vi "Initialize Sink.vi"(11 "Buffered Log Sink in":refnum<class "Buffered Log Sink.lvclass">) -> (0 "error out":errorcluster, 3 "Buffered Log Sink out":refnum<class "Buffered Log Sink.lvclass">)   [LabVIEW 2020, in "Buffered Log Sink.lvclass"]
uses:
  <vilib>/gpm_packages/@cs/event-logger/Source/Buffered Log Sink/Buffered Log Sink.lvclass
  <vilib>/gpm_packages/@cs/event-logger/Source/Buffered Log Sink/Buffered Log Sink.lvclass/Buffered Log Sink.ctl
  <vilib>/gpm_packages/@cs/event-logger/Source/Composed Log/Types/Log Packet.ctl
  <vilib>/gpm_packages/@cs/event-logger/Source/Composed Log/Types/Log Level.ctl
  <vilib>/gpm_packages/@cs/event-logger/Source/Buffered Log Sink/Timeout Watchdog.vi
  <vilib>/gpm_packages/@cs/event-logger/Source/Composed Log/Log Sink/Log Sink.lvclass
  <vilib>/gpm_packages/@cs/event-logger/Source/Composed Log/Composed Log.lvlib
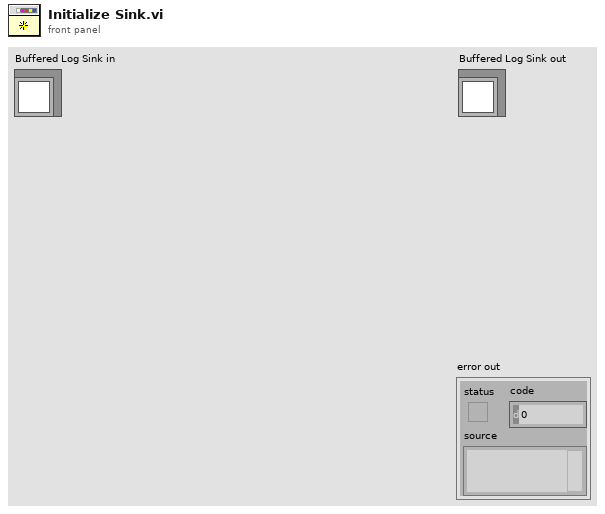
[diagram p1: front panel]
types:
  T1 = typedef "Composed Log.lvlib/Log Packet.ctl" = cluster{"Data To Log":string, "Source":string, "Event Level":T2, "Event Time":timestamp}
  T2 = typedef "Composed Log.lvlib/Log Level.ctl" = enum16{"Debug", "Info", "Warning", "Error", "Critical"}
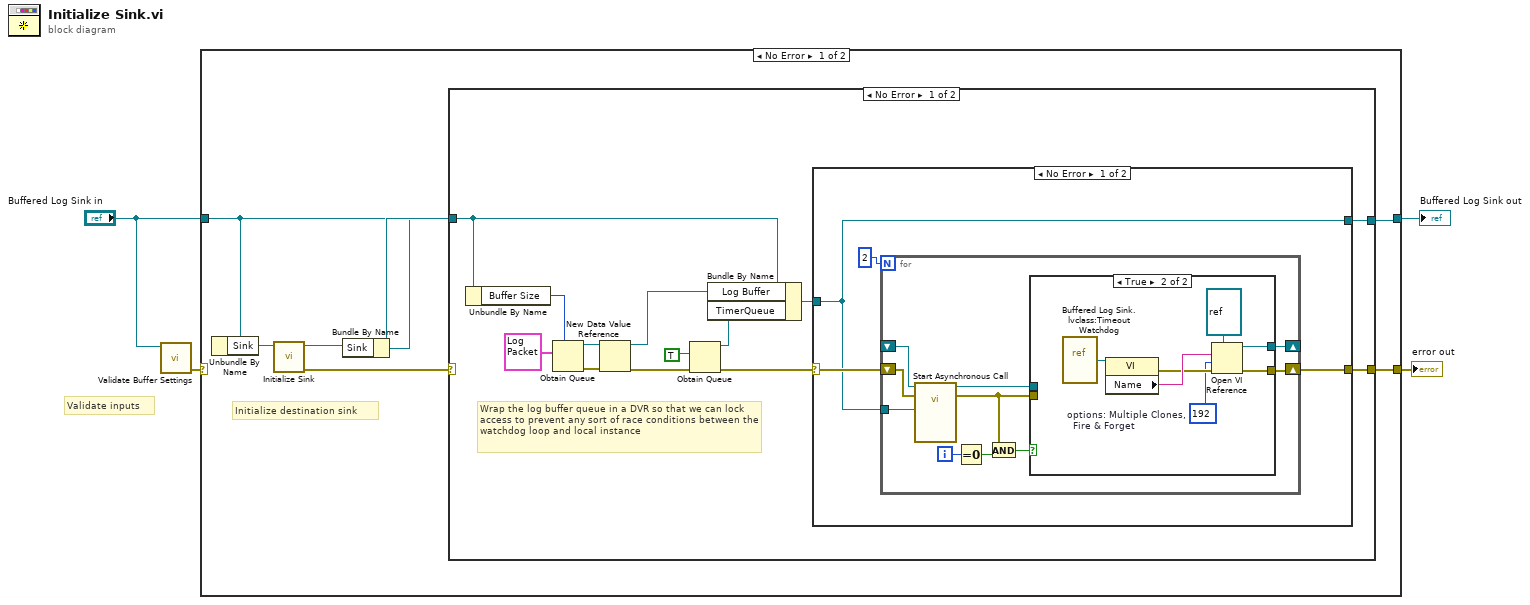
[diagram p0: block diagram]
diagram:
  # "Validate inputs"
  n1 = call <vilib>:"Validate Buffer Settings.vi"("Buffered Log Sink in"="Buffered Log Sink in") -> ("error out"=w1:errorcluster)  [unwired: 10 in]
  n2 = case shown="No Error" w1 {
    selector: w1 -> [_ w52]
    tunnel: [w11 w53] -> w4
    tunnel: [w10 w52] -> w3
    tunnel: "Buffered Log Sink in" -> [w8 w53]
    frame No Error {
      # "Initialize destination sink"
      n3 = Unbundle By Name(w8) -> ("Sink"=w7:refnum<class "Log Sink.lvclass">)
      n4 = call-dynamic "Initialize Sink.vi"("Log Sink in"=w7) -> ("error out"=w6:errorcluster, "Log Sink out"=w5:refnum<class "Log Sink.lvclass">)  [unwired: 9 in]
      n5 = Bundle By Name(cluster=w8, "Sink"=w5) -> (w9:refnum<class "Buffered Log Sink.lvclass">)
      n6 = case shown="No Error" w6 {
        selector: w6 -> [_ w50]
        tunnel: [w14 w51] -> w11
        tunnel: [w13 w50] -> w10
        tunnel: w9 -> [w12 w51]
        frame No Error {
          # "Wrap the log buffer queue in a DVR so that we can lock access to prevent any sort of race conditions between the watchdog loop and local instance"
          n7 = Unbundle By Name(w12) -> ("Buffer Size"=w18:i32)
          n8 = Obtain Queue(max queue size (-1, unlimited)=w18, element data type=T1 {"Data To Log"="", "Source"="", "Event Level"=enum."Debug", "Event Time"=timestamp(0 s since 1904-01-01)} ("Log Packet")) -> (queue out=w20:refnum<queue>, error out=w17:errorcluster)  [unwired: 3 in, 1 out]
          n9 = New Data Value Reference(data value=w20, error in=w17) -> (data value reference=w19:refnum<data-value>, error out=w16:errorcluster)
          n10 = Obtain Queue(element data type=TRUE, error in (no error)=w16) -> (queue out=w21:refnum<queue>, error out=w15:errorcluster)  [unwired: 3 in, 1 out]
          n11 = Bundle By Name(cluster=w12, "Log Buffer"=w19, "TimerQueue"=w21) -> (w22:refnum<class "Buffered Log Sink.lvclass">)
          n12 = case shown="No Error" w15 {
            selector: w15 -> [w27 w48]
            tunnel: w22 -> [w26 w49]
            tunnel: [w26 w49] -> w14
            tunnel: [w25 w48] -> w13
            frame No Error {
              n13 = for {
                N: 2 -> [_]
                shift-right: [w34] -> _
                shift-left: _ -> [w38]
                tunnel: w26 -> [w30]
                shift-right: [w32] -> w25
                shift-left: w27 -> [w29]
                i -> [w37]
                n14 = call-by-ref "Start Asynchronous Call"(reference=w38, error in=w29, "Buffered Log Sink in"=w30) -> (reference out=w35:refnum<vi>, error out=w31:errorcluster)  [unwired: 11 in]
                n15 = Equal To 0?(x=w37) -> (x = 0?=w36:bool)
                n16 = And(x=w31, y=w36) -> (x .and. y?=w33:bool)
                n17 = case shown="True" w33 {
                  tunnel: w35 -> [w40 _]
                  tunnel: [w39 w43] -> w32
                  tunnel: [w40 w42] -> w34
                  tunnel: w31 -> [w39 _]
                  frame False {
                  }
                  frame True {
                    w41 = 192  # options: Multiple Clones,   Fire & Forget
                    n18 = vi-ref "Buffered Log Sink.lvclass:Timeout Watchdog.vi"() -> (w45:refnum<vi>)
                    n19 = property class="VI"(reference=w45) -> (error out=w46:errorcluster, "Name"=w47:string)  [unwired: 1 in, 1 out]
                    n20 = Open VI Reference(type specifier VI Refnum (for type only)=refnum<vi> refnum, vi path=w47, options=w41, error in (no error)=w46) -> (vi reference=w42:refnum<vi>, error out=w43:errorcluster)  [unwired: 2 in]
                  }
                }
              }
            }
            frame Error {
            }
          }
        }
        frame Error {
        }
      }
    }
    frame Error {
      # "Invalid buffer settings"
    }
  }
  "error out" <- w3
  "Buffered Log Sink out" <- w4
